vi "Dispense.vi"(8 "error in (no error)":errorcluster, 10 "BallsIn":i32, 11 "object in":refnum<class "NoMoneyState.lvclass">) -> (0 "error out":errorcluster, 2 "BallsOut":i32, 3 "object out":refnum<class "State.lvclass">)   [LabVIEW 2020, in "NoMoneyState.lvclass"]
uses:
  NoMoneyState.lvclass
  C:/Projects/OpenGDS_DesignPatterns/State1/State_class/State.lvclass
  State_class/State.lvclass
  NoMoneyState.lvclass/NoMoneyState.ctl
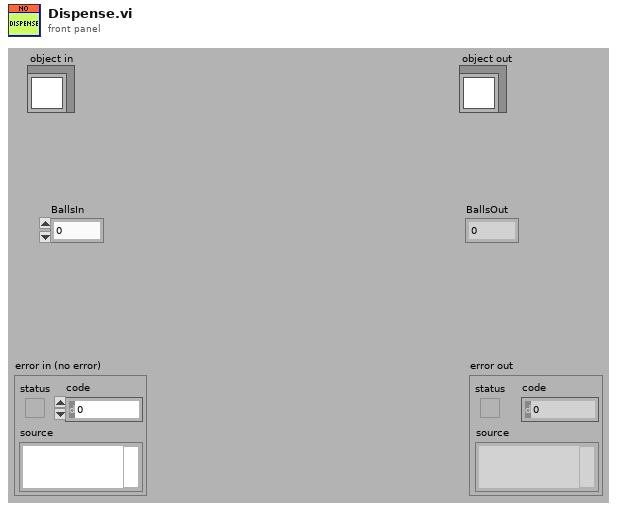
[diagram p1: front panel]
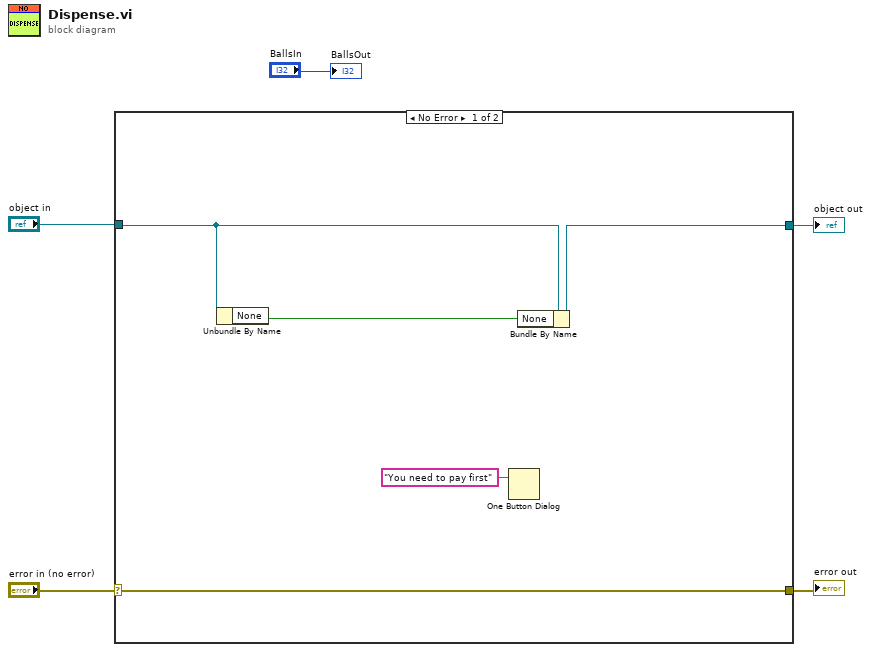
[diagram p0: block diagram]
diagram:
  n1 = case shown="No Error" "error in (no error)" {
    selector: "error in (no error)" -> [w9 w12]
    tunnel: [w9 w12] -> w4
    tunnel: [w7 w11] -> w2
    tunnel: "object in" -> [w8 w11]
    frame No Error {
      n2 = Unbundle By Name(w8) -> ("None"=w10:bool)
      n3 = One Button Dialog(message="You need to pay first" ("TextIn")) -> ()  [unwired: 1 in, 1 out]
      n4 = Bundle By Name(cluster=w8, "None"=w10) -> (w7:refnum<class "NoMoneyState.lvclass">)
    }
    frame Error {
    }
  }
  "error out" <- w4
  "object out" <- w2
  "BallsOut" <- "BallsIn"
